vi "Flush FPGA Queue.vi"(8 "error in":errorcluster, 11 "Refnum in":T1) -> (0 "error out":errorcluster)   [LabVIEW 2017, in "gCRDS.lvlib" / "gCRD.lvclass"]
uses:
  gCRD.lvclass
  FPGA Ref.ctl
  <vilib>/Utility/error.llb/Error Cluster From Error Code.vi
  <vilib>/rvi/errors/niLvFpgaAdjustHostInterfaceError.vi
  <vilib>/rvi/interface/nirviReadWriteControl/nirviReadWriteControl.xnode
  FPGA Bitfiles/server.lvbitx
  <vilib>/rvi/interface/nirviMethod/nirviMethod.xnode
  NiFpgaLv.dll
  <vilib>/FPGAPlugInAG/cRIO-9081/niLvFpga_ReadFifo_cRIO-9081.vi
  <vilib>/rvi/errors/niLvFpgaMergeErrorWithErrorCode.vi
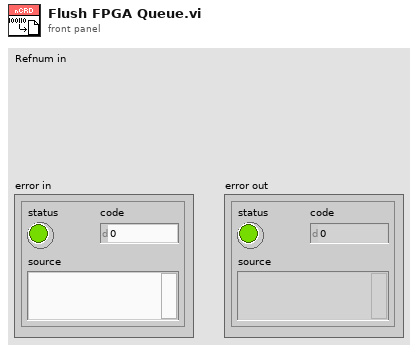
[diagram p1: front panel]
types:
  T1 = typedef "FPGA Ref.ctl" = refnum<k20>
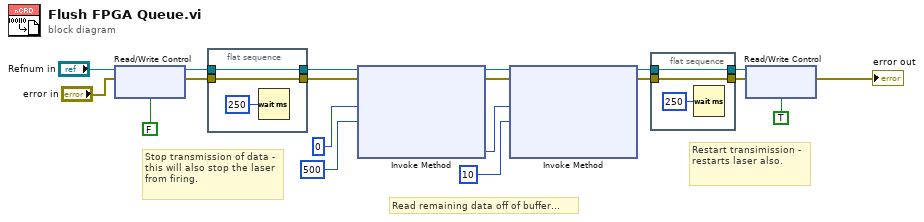
[diagram p0: block diagram]
diagram:
  # "Restart transimission - restarts laser also."
  # "Stop transmission of data - this will also stop the laser from firing."
  # "Read remaining data off of buffer..."
  n1 = xnode "Read/Write Control"("FPGA VI Reference In"="Refnum in", "error in"="error in", "Transmit?"=FALSE) -> ("FPGA VI Reference Out"=w13:T1, "error out"=w15:errorcluster)
  n2 = flat-sequence {
    tunnel: w13 -> [w21]
    tunnel: [w21] -> w14
    tunnel: [w20] -> w16
    tunnel: w15 -> [w20]
    frame #0 {
      n3 = Wait (ms)(milliseconds to wait=u32 250) -> ()  [unwired: 1 out]
    }
  }
  n4 = xnode "Invoke Method"("FPGA VI Reference In"=w14, "error in"=w16, "Number of Elements"=u32 0, "Timeout (ms)"=500) -> ("FPGA VI Reference Out"=w7:T1, "error out"=w6:errorcluster, "Elements Remaining"=w10:u32)  [unwired: 1 out]
  n5 = xnode "Invoke Method"("FPGA VI Reference In"=w7, "error in"=w6, "Number of Elements"=w10, "Timeout (ms)"=10) -> ("FPGA VI Reference Out"=w18:T1, "error out"=w9:errorcluster)  [unwired: 2 out]
  n6 = flat-sequence {
    tunnel: w9 -> [w24]
    tunnel: [w24] -> w8
    tunnel: w18 -> [w23]
    tunnel: [w23] -> w19
    frame #0 {
      n7 = Wait (ms)(milliseconds to wait=u32 250) -> ()  [unwired: 1 out]
    }
  }
  n8 = xnode "Read/Write Control"("FPGA VI Reference In"=w19, "error in"=w8, "Transmit?"=TRUE) -> ("error out"=→"error out":errorcluster)  [unwired: 1 out]
